vi "PicoLogStart.vi"(1 "sampleInterval_ms":i32=1000, 2 "conversionTime":i16(ring) items=["60 ms", "100 ms", "180 ms", "340 ms", "660 ms"], 3 "Mains Frequency":i16(ring) items=["50 Hz", "60 Hz"], 9 "4":bool, 11 "5":bool) -> (12 "noOfChannels":i16=2, 13 "STOP":bool, 14 "handle":i16)   [LabVIEW 2014]
uses:
  Instance           1 22Saved   HRDL_streaming .vi
  Instance         138 22Saved   HRDL_streaming .vi
  picohrdl.dll
panel:
  in  "Voltage range":i32[](array[numeric]) min=0 max=6 step=1
  in  "Single ended\n(0- single)\n(1 - difer)":i32[](array[numeric]) min=0 max=1 step=1
  in  "Ch nr":bool[](array[boolean])
  out "Unit Info":T1
  in  "13":bool
  in  "12":bool
  in  "11":bool
  in  "10":bool
  in  "9":bool
  in  "8":bool
  in  "7":bool
  in  "6":bool
  # "1       2       3      4       5        6       7       8       9      10     11      12     13    14       15     16"
  # "0 -+2500mV\n1 -+1250mV\n2 -+625mV\n3 -+313mV\n4 -+156mV\n5 -+78mv\n6 -+39mV"
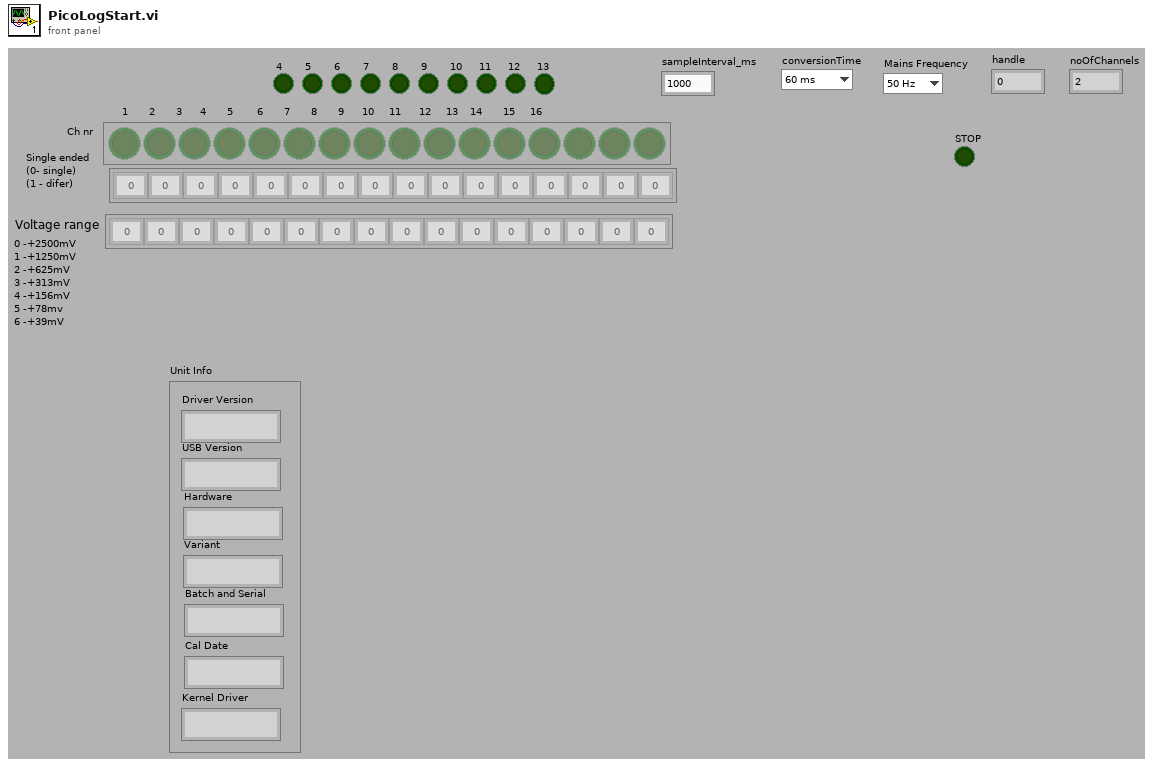
[diagram p1: front panel]
types:
  T1 = cluster{"Driver Version":string, "USB Version":string, "Hardware":string, "Variant":string, "Batch and Serial":string, "Cal Date":string, "Kernel Driver":string}
  T2 = cluster{"[0]":string, "[1]":string, "[2]":string, "[3]":string, "[4]":string, "[5]":string, "[6]":string}
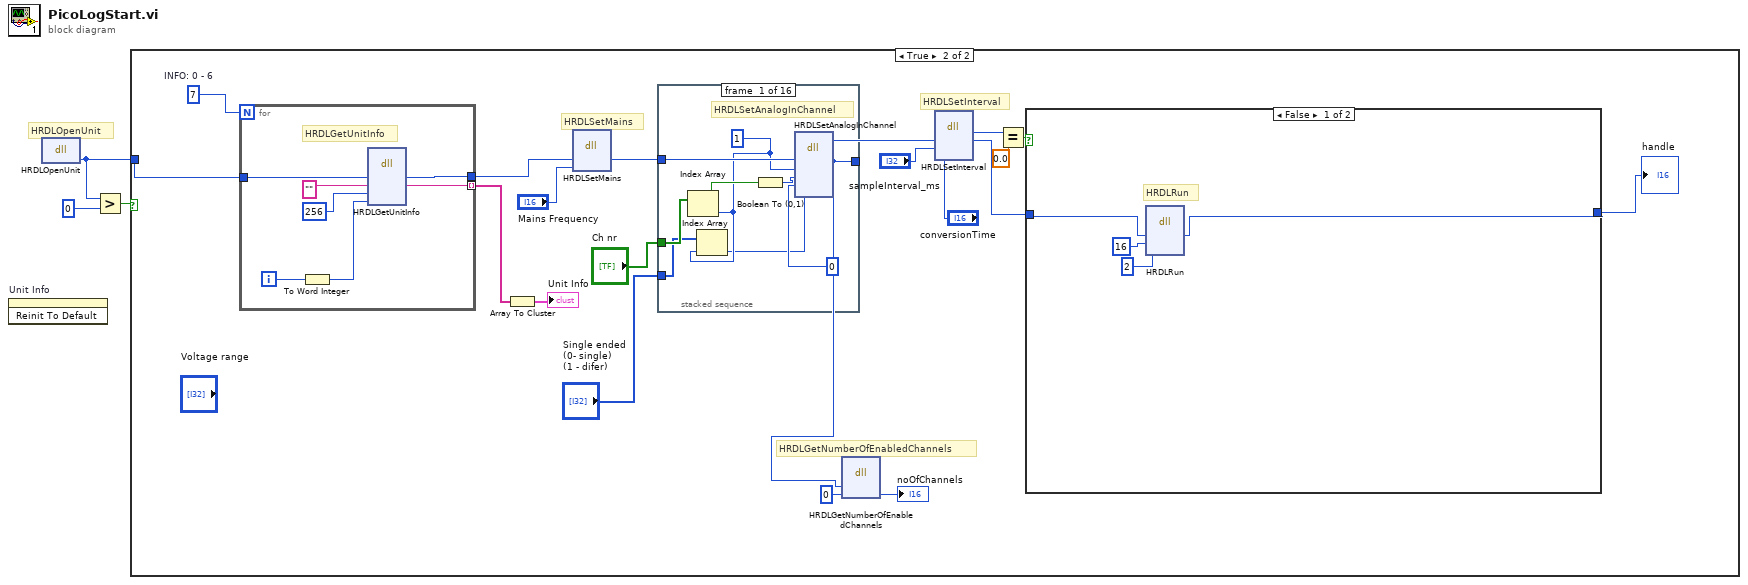
[diagram p0: block diagram]
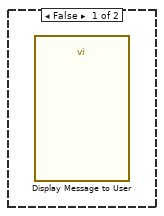
[diagram p2: hidden frame]
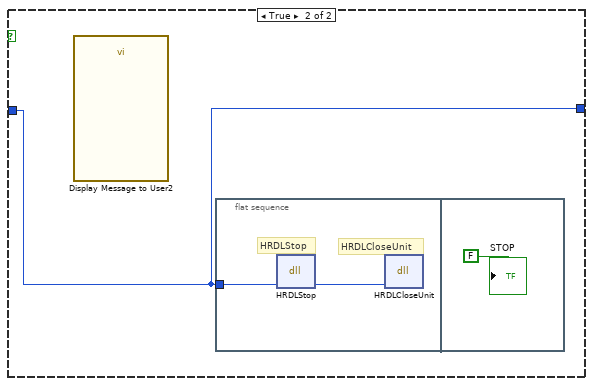
[diagram p3: hidden frame]
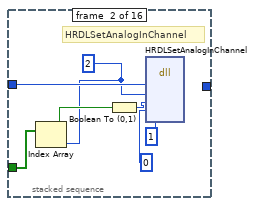
[diagram p4: hidden frame]
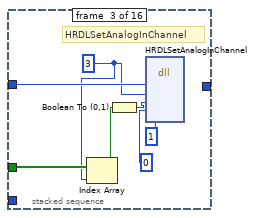
[diagram p5: hidden frame]
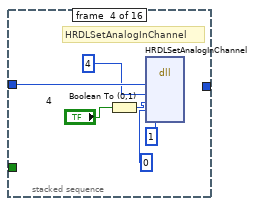
[diagram p6: hidden frame]
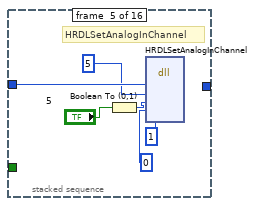
[diagram p7: hidden frame]
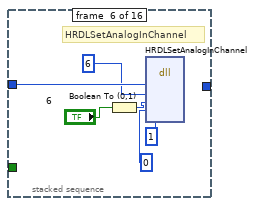
[diagram p8: hidden frame]
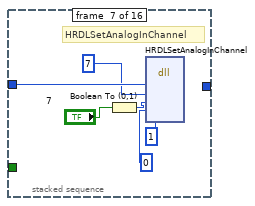
[diagram p9: hidden frame]
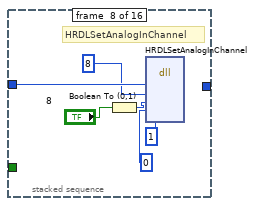
[diagram p10: hidden frame]
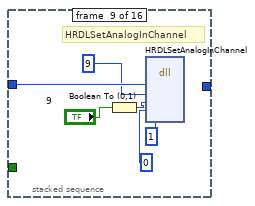
[diagram p11: hidden frame]
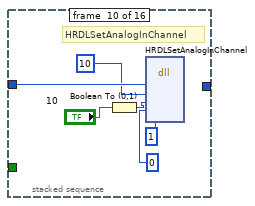
[diagram p12: hidden frame]
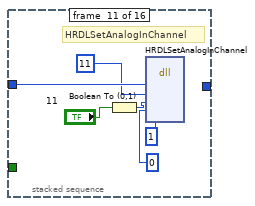
[diagram p13: hidden frame]
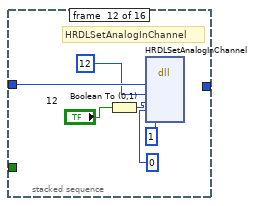
[diagram p14: hidden frame]
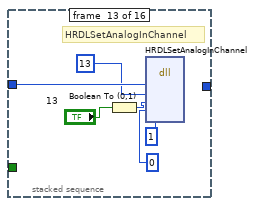
[diagram p15: hidden frame]
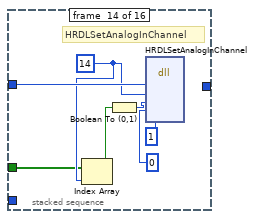
[diagram p16: hidden frame]
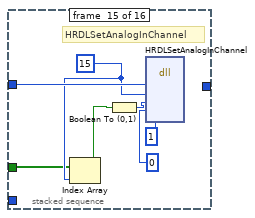
[diagram p17: hidden frame]
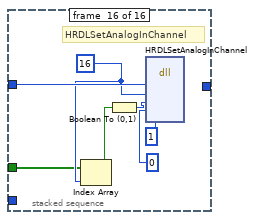
[diagram p18: hidden frame]
diagram:
  # "HRDLOpenUnit"
  n1 = invoke on="Unit Info" class="Clust (strict)" method="Reinit To Default"() -> ()  [unwired: 3 in, 3 out]
  n2 = dll-call lib="picohrdl.dll" fn="HRDLOpenUnit"() -> ("handle"=w1:i16)  [unwired: 3 in, 2 out]
  n3 = Greater?(x=w1, y=i16 0) -> (0:w3:bool)
  n4 = case shown="True" w3 {
    tunnel: w1 -> [_ w11]
    frame False {
      n5 = call "Display Message to User"() -> ()  [unwired: 10 in, 2 out]
    }
    frame True {
      w13 = 7  # INFO: 0 - 6
      # "HRDLGetNumberOfEnabledChannels"
      # "HRDLSetInterval"
      # "HRDLSetMains"
      n6 = for {
        N: w13 -> [_]
        tunnel: w11 -> [w29]
        tunnel: [w26] -> w10 mode=indexing
        tunnel: [w24] -> w12
        i -> [w25]
        # "HRDLGetUnitInfo"
        n7 = To Word Integer(number=w25) -> (16bit integer=w23:i16)
        n8 = dll-call lib="picohrdl.dll" fn="HRDLGetUnitInfo"("handle"=w29, "unitInfo"="", "stringLength"=i16 256, "info"=w23) -> ("handle"=w24:i16, "unitInfo"=w26:string)  [unwired: 6 in, 2 out]
      }
      n9 = Array To Cluster(array=w10) -> (cluster=→"Unit Info":T2)
      n10 = dll-call lib="PicoHRDL.dll" fn="HRDLSetMains"("handle"=w12, "sixtyHertz"="Mains Frequency") -> ("handle"=w15:i16)  [unwired: 5 in, 2 out]
      n11 = stacked-sequence {
        tunnel: w15 -> [w46 w53 w60 w66 w72 w78 w84 w90 w96 w102 w108 w114 w120 w127 w134 w141]
        tunnel: [w45 _ _ _ _ _ _ _ _ _ _ _ _ _ _ _] -> w14
        tunnel: "Ch nr" -> [w42 w49 w55 _ _ _ _ _ _ _ _ _ _ w121 w128 w135]
        tunnel: "Single ended\n(0- single)\n(1 - difer)" -> [w40 _ _ _ _ _ _ _ _ _ _ _ _ _ _ _]
        frame #0 {
          w39 = i16 1 ("channel")
          # "HRDLSetAnalogInChannel"
          n12 = Index Array(array=w42, index=w39) -> (element=w41:bool)
          n13 = Index Array(array=w40, index=w39) -> (element=w38:i32)
          n14 = Boolean To (0,1)(Boolean=w41) -> (0, 1=w43:i16)
          n15 = dll-call lib="PicoHRDL.dll" fn="HRDLSetAnalogInChannel"("handle"=w46, "channel"=w39, "enabled"=w43, "range"=i16 0 ("range 1"), "singleEnded"=w38) -> ("handle"=w45:i16)  [unwired: 8 in, 2 out]
        }
        frame #1 {
          w47 = i16 2 ("channel")
          # "HRDLSetAnalogInChannel"
          n16 = Index Array(array=w49, index=w47) -> (element=w48:bool)
          n17 = Boolean To (0,1)(Boolean=w48) -> (0, 1=w50:i16)
          n18 = dll-call lib="PicoHRDL.dll" fn="HRDLSetAnalogInChannel"("handle"=w53, "channel"=w47, "enabled"=w50, "range"=i16 0 ("range 2"), "singleEnded"=i16 1) -> ()  [unwired: 9 in, 2 out]
        }
        frame #2 {
          w54 = i16 3 ("channel")
          # "HRDLSetAnalogInChannel"
          n19 = Index Array(array=w55, index=w54) -> (element=w56:bool)
          n20 = Boolean To (0,1)(Boolean=w56) -> (0, 1=w57:i16)
          n21 = dll-call lib="PicoHRDL.dll" fn="HRDLSetAnalogInChannel"("handle"=w60, "channel"=w54, "enabled"=w57, "range"=i16 0 ("range 3"), "singleEnded"=i16 1) -> ()  [unwired: 9 in, 2 out]
        }
        frame #3 {
          # "HRDLSetAnalogInChannel"
          n22 = Boolean To (0,1)(Boolean="4") -> (0, 1=w62:i16)
          n23 = dll-call lib="PicoHRDL.dll" fn="HRDLSetAnalogInChannel"("handle"=w66, "channel"=i16 4, "enabled"=w62, "range"=i16 0 ("range 4"), "singleEnded"=i16 1) -> ()  [unwired: 9 in, 2 out]
        }
        frame #4 {
          # "HRDLSetAnalogInChannel"
          n24 = Boolean To (0,1)(Boolean="5") -> (0, 1=w68:i16)
          n25 = dll-call lib="PicoHRDL.dll" fn="HRDLSetAnalogInChannel"("handle"=w72, "channel"=i16 5, "enabled"=w68, "range"=i16 0 ("range 5"), "singleEnded"=i16 1) -> ()  [unwired: 9 in, 2 out]
        }
        frame #5 {
          # "HRDLSetAnalogInChannel"
          n26 = Boolean To (0,1)(Boolean="6") -> (0, 1=w74:i16)
          n27 = dll-call lib="PicoHRDL.dll" fn="HRDLSetAnalogInChannel"("handle"=w78, "channel"=i16 6, "enabled"=w74, "range"=i16 0 ("range 6"), "singleEnded"=i16 1) -> ()  [unwired: 9 in, 2 out]
        }
        frame #6 {
          # "HRDLSetAnalogInChannel"
          n28 = Boolean To (0,1)(Boolean="7") -> (0, 1=w80:i16)
          n29 = dll-call lib="PicoHRDL.dll" fn="HRDLSetAnalogInChannel"("handle"=w84, "channel"=i16 7, "enabled"=w80, "range"=i16 0 ("range 7"), "singleEnded"=i16 1) -> ()  [unwired: 9 in, 2 out]
        }
        frame #7 {
          # "HRDLSetAnalogInChannel"
          n30 = Boolean To (0,1)(Boolean="8") -> (0, 1=w86:i16)
          n31 = dll-call lib="PicoHRDL.dll" fn="HRDLSetAnalogInChannel"("handle"=w90, "channel"=i16 8, "enabled"=w86, "range"=i16 0 ("range 8"), "singleEnded"=i16 1) -> ()  [unwired: 9 in, 2 out]
        }
        frame #8 {
          # "HRDLSetAnalogInChannel"
          n32 = Boolean To (0,1)(Boolean="9") -> (0, 1=w92:i16)
          n33 = dll-call lib="PicoHRDL.dll" fn="HRDLSetAnalogInChannel"("handle"=w96, "channel"=i16 9, "enabled"=w92, "range"=i16 0 ("range 9"), "singleEnded"=i16 1) -> ()  [unwired: 9 in, 2 out]
        }
        frame #9 {
          # "HRDLSetAnalogInChannel"
          n34 = Boolean To (0,1)(Boolean="10") -> (0, 1=w98:i16)
          n35 = dll-call lib="PicoHRDL.dll" fn="HRDLSetAnalogInChannel"("handle"=w102, "channel"=i16 10, "enabled"=w98, "range"=i16 0 ("range 10"), "singleEnded"=i16 1) -> ()  [unwired: 9 in, 2 out]
        }
        frame #10 {
          # "HRDLSetAnalogInChannel"
          n36 = Boolean To (0,1)(Boolean="11") -> (0, 1=w104:i16)
          n37 = dll-call lib="PicoHRDL.dll" fn="HRDLSetAnalogInChannel"("handle"=w108, "channel"=i16 11, "enabled"=w104, "range"=i16 0 ("range 11"), "singleEnded"=i16 1) -> ()  [unwired: 9 in, 2 out]
        }
        frame #11 {
          # "HRDLSetAnalogInChannel"
          n38 = Boolean To (0,1)(Boolean="12") -> (0, 1=w110:i16)
          n39 = dll-call lib="PicoHRDL.dll" fn="HRDLSetAnalogInChannel"("handle"=w114, "channel"=i16 12, "enabled"=w110, "range"=i16 0 ("range 12"), "singleEnded"=i16 1) -> ()  [unwired: 9 in, 2 out]
        }
        frame #12 {
          # "HRDLSetAnalogInChannel"
          n40 = Boolean To (0,1)(Boolean="13") -> (0, 1=w116:i16)
          n41 = dll-call lib="PicoHRDL.dll" fn="HRDLSetAnalogInChannel"("handle"=w120, "channel"=i16 13, "enabled"=w116, "range"=i16 0 ("range 13"), "singleEnded"=i16 1) -> ()  [unwired: 9 in, 2 out]
        }
        frame #13 {
          w122 = i16 14 ("channel")
          # "HRDLSetAnalogInChannel"
          n42 = Index Array(array=w121, index=w122) -> (element=w123:bool)
          n43 = Boolean To (0,1)(Boolean=w123) -> (0, 1=w124:i16)
          n44 = dll-call lib="PicoHRDL.dll" fn="HRDLSetAnalogInChannel"("handle"=w127, "channel"=w122, "enabled"=w124, "range"=i16 0 ("range 14"), "singleEnded"=i16 1) -> ()  [unwired: 9 in, 2 out]
        }
        frame #14 {
          w129 = i16 15 ("channel")
          # "HRDLSetAnalogInChannel"
          n45 = Index Array(array=w128, index=w129) -> (element=w130:bool)
          n46 = Boolean To (0,1)(Boolean=w130) -> (0, 1=w131:i16)
          n47 = dll-call lib="PicoHRDL.dll" fn="HRDLSetAnalogInChannel"("handle"=w134, "channel"=w129, "enabled"=w131, "range"=i16 0 ("range 15"), "singleEnded"=i16 1) -> ()  [unwired: 9 in, 2 out]
        }
        frame #15 {
          w136 = i16 16 ("channel")
          # "HRDLSetAnalogInChannel"
          n48 = Index Array(array=w135, index=w136) -> (element=w137:bool)
          n49 = Boolean To (0,1)(Boolean=w137) -> (0, 1=w138:i16)
          n50 = dll-call lib="PicoHRDL.dll" fn="HRDLSetAnalogInChannel"("handle"=w141, "channel"=w136, "enabled"=w138, "range"=i16 0 ("range 16"), "singleEnded"=i16 1) -> ()  [unwired: 9 in, 2 out]
        }
      }
      n51 = dll-call lib="PicoHRDL.dll" fn="HRDLGetNumberOfEnabledChannels"("handle"=w14, "nEnabledChannels"=i16 0) -> ("nEnabledChannels"=→"noOfChannels":i16)  [unwired: 5 in, 2 out]
      n52 = dll-call lib="PicoHRDL.dll" fn="HRDLSetInterval"("handle"=w14, "sampleInterval_ms"="sampleInterval_ms", "conversionTime"="conversionTime") -> ("return type"=w19:i16, "handle"=w18:i16)  [unwired: 5 in, 2 out]
      n53 = Equal?(x=w19, y=0.0) -> (x = y?=w17:bool)
      n54 = case shown="False" w17 {
        tunnel: [w30 w34] -> w8
        tunnel: w18 -> [w31 w34]
        frame False {
          # "HRDLRun"
          n55 = dll-call lib="PicoHRDL.dll" fn="HRDLRun"("handle"=w31, "nValues"=16, "method"=i16 2) -> ("handle"=w30:i16)  [unwired: 6 in, 2 out]
        }
        frame True {
          n56 = call "Display Message to User2"() -> ()  [unwired: 10 in, 2 out]
          n57 = flat-sequence {
            tunnel: w34 -> [w35]
            frame #0 {
              # "HRDLStop"
              # "HRDLCloseUnit"
              n58 = dll-call lib="picohrdl.dll" fn="HRDLStop"("handle"=w35) -> ("handle"=w36:i16)  [unwired: 4 in, 2 out]
              n59 = dll-call lib="PicoHRDL.dll" fn="HRDLCloseUnit"("handle"=w36) -> ()  [unwired: 5 in, 2 out]
            }
            frame #1 {
              "STOP" <- FALSE ("stop")
            }
          }
        }
      }
      "handle" <- w8
    }
  }
